vi "Get Item with CH# from section.vi"(8 "error in (no error)":errorcluster, 9 "CH#":i32, 10 "Section containing ch#":string, 11 "Item Ref in":T1 format="%.0x") -> (0 "error out":errorcluster, 2 "Matching CH# item in Specified Section":T1 format="%.0x", 3 "Item Ref out":T1 format="%.0x", 4 "Found":bool)   [LabVIEW 2011, in "NI 272x Resistive Simulation Custom Device Configuration.lvlib"]
uses:
  NI 272x Resistive Simulation Custom Device Configuration.lvlib
  <vilib>/NI Veristand/Custom Device API/Custom Device Item Ref.ctl
  <vilib>/NI Veristand/Custom Device Tools/Custom Device Utility Library/Search Direction.ctl
  Globals/Names.vi
  <vilib>/NI Veristand/Custom Device Tools/Custom Device Utility Library/NI VeriStand - Search for Item by GUID.vi
  <vilib>/NI Veristand/Custom Device Tools/Custom Device Utility Library/NI VeriStand - Search for Item by Name.vi
  <vilib>/NI Veristand/Custom Device Tools/Custom Device Utility Library/NI VeriStand - Search for Item by Property.vi
  <vilib>/NI Veristand/Custom Device Tools/Custom Device Utility Library/Custom Device Utility Library.lvlib
  NI 272x Resistive Simulation Custom Device Shared.lvlib
  <vilib>/NI Veristand/Custom Device API/Custom Device API.lvlib
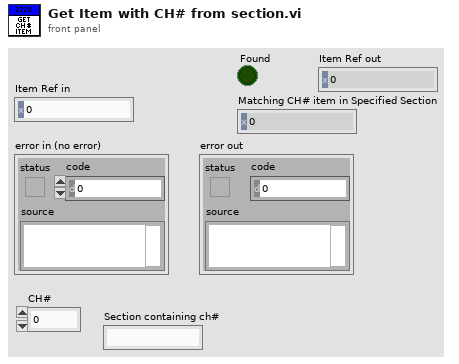
[diagram p1: front panel]
types:
  T1 = typedef "Custom Device API.lvlib/Custom Device Item Ref.ctl" = u64
  T2 = typedef "Custom Device Utility Library.lvlib/Search Direction.ctl" = enum16{"Down", "Up"}
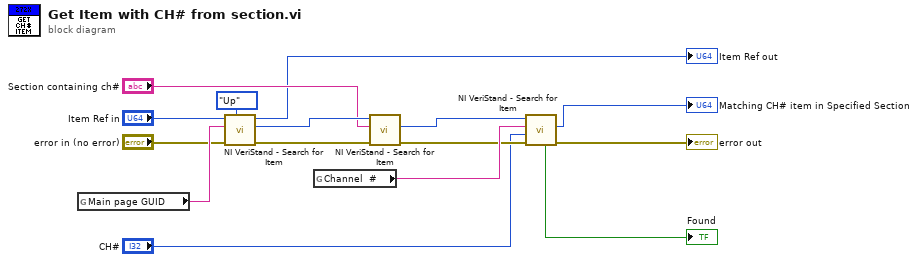
[diagram p0: block diagram]
diagram:
  n1 = global read "Names.vi" "Main page GUID"() -> (w14:string)
  n2 = call-poly <vilib>:"NI VeriStand - Search for Item.vi"("Direction (Down)"=Search_Direction."Up", "error in"="error in (no error)", "Item GUID"=w14, "Section Ref in"="Item Ref in") -> ("error out"=w9:errorcluster, "Item Ref"=w13:T1, "Section Ref out"=→"Item Ref out":T1)  [unwired: 4 in, 1 out]
  n3 = global read "Names.vi" "Channel  #"() -> (w7:string)
  n4 = call-poly <vilib>:"NI VeriStand - Search for Item.vi"("error in"=w9, "Item Name"="Section containing ch#", "Section Ref in"=w13) -> ("error out"=w6:errorcluster, "Item Ref"=w5:T1)  [unwired: 5 in, 2 out]
  n5 = call-poly <vilib>:"NI VeriStand - Search for Item.vi"("error in"=w6, "Property Value"="CH#", "Property Name"=w7, "Section Ref in"=w5) -> ("error out"=→"error out":errorcluster, "Item Ref"=→"Matching CH# item in Specified Section":T1, "Found"=→"Found":bool)  [unwired: 4 in, 1 out]
